vi "ThrowError.vi"(8 "error in (no error)":errorcluster, 9 "type of dialog (OK msg:1)":T1=1 items=["no dialog", "OK message", "continue or stop message", "OK message + warnings", "continue/stop + warnings"], 10 "Error Message":string="Default Error Message!", 11 "Error Input":bool=TRUE) -> (0 "error out":errorcluster, 3 "Error Input Passthrough":bool)   [LabVIEW 2013]
uses:
  <vilib>/Utility/error.llb/DialogType.ctl
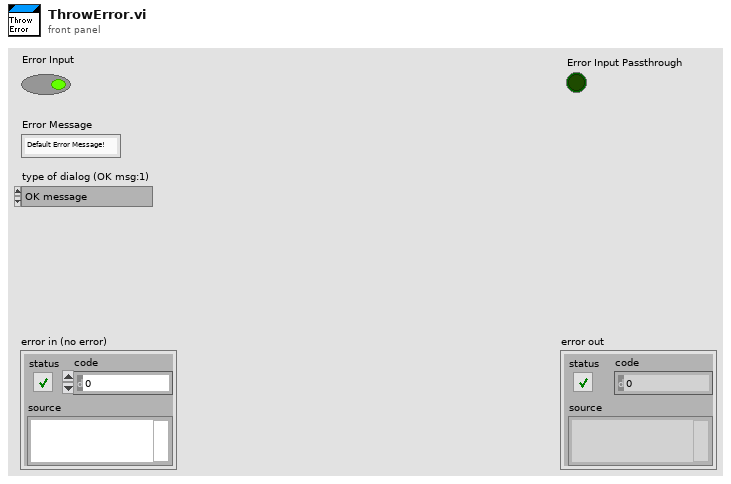
[diagram p1: front panel]
types:
  T1 = typedef "DialogType.ctl" = u16
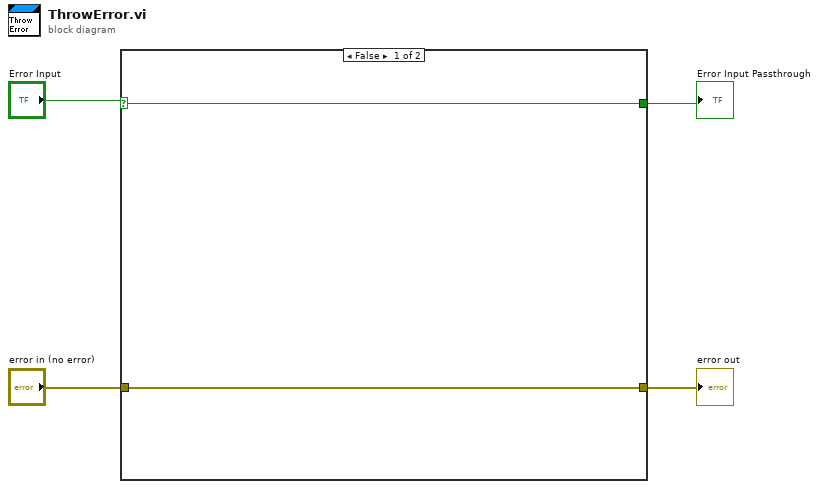
[diagram p0: block diagram]
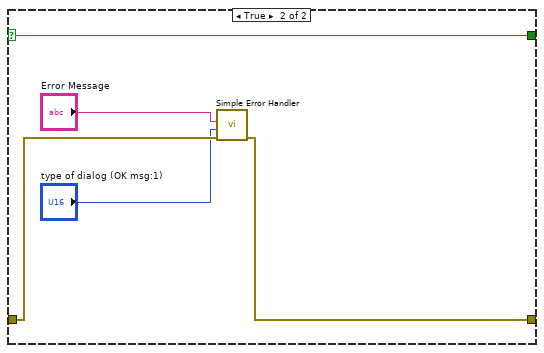
[diagram p2: hidden frame]
diagram:
  n1 = case shown="False" "Error Input" {
    selector: "Error Input" -> [w6 w11]
    tunnel: [w6 w11] -> w3
    tunnel: "error in (no error)" -> [w5 w10]
    tunnel: [w5 w9] -> w1
    frame False {
    }
    frame True {
      n2 = call <vilib>:"Simple Error Handler.vi"("error source (\" \")"="Error Message", "type of dialog (OK msg:1)"="type of dialog (OK msg:1)", "error in (no error)"=w10) -> ("error out"=w9:errorcluster)  [unwired: 2 in, 4 out]
    }
  }
  "error out" <- w1
  "Error Input Passthrough" <- w3
